vi "3 - Basic Measurement (Solution).vi"() -> ()   [LabVIEW 2013]
panel:
  out "Temperature Data":dynamicdata(graph)
  in  "stop":bool
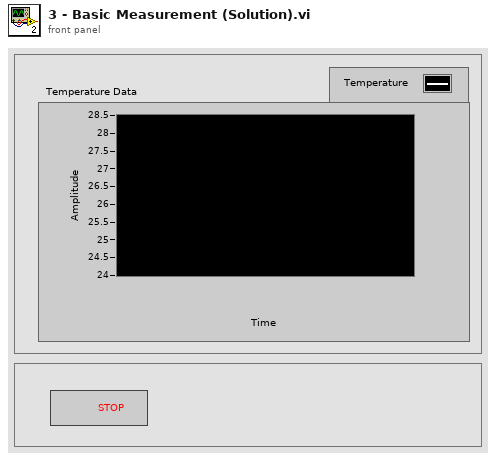
[diagram p1: front panel]
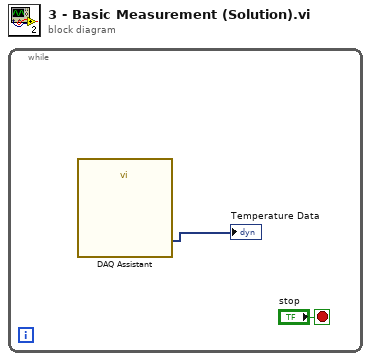
[diagram p0: block diagram]
diagram:
  n1 = while {
    stop <- "stop" stop-if-true
    n2 = call "DAQ Assistant"() -> ("data"=→"Temperature Data":dynamicdata)  [unwired: 16 in, 3 out]
  }
